vi "Associate Instruments to Paths.vi"(0 "Vector Path Group in":refnum<class "Vector Path Group.lvclass">, 5 "TSM Context":T1, 11 "error in (no error)":errorcluster) -> (4 "Vector Path Group out":refnum<class "Vector Path Group.lvclass">, 15 "error out":errorcluster)   [LabVIEW 2023, in "RFFixtureCharact.Public.lvlib" / "Vector Path Group.lvclass"]
uses:
  Vector Path Group.lvclass
  C:/rfcal/AuxTools/STSRFFixtureCharactUtility/Source/Code Modules/Common/Base Classes/Path Group/Path Group.lvclass
  <vilib>/NI_TestStand_SemiconductorModule/NI_TestStand_Semiconductor_Module.lvlibp/PinMap/General/SemiconductorModuleContext.ctl
  Instruments/Cal Standard/Cal Standard Base/Cal Standard Base.lvclass/Cal Standard Base.ctl
  Charact Result Accessor/Vector/Vector Charact Result Accessor.lvclass
  C:/rfcal/AuxTools/STSRFFixtureCharactUtility/Source/Code Modules/Fixture/Public/Charact Result Accessor/Base/Charact Result Accessor.lvclass
  C:/rfcal/AuxTools/STSRFFixtureCharactUtility/Source/Code Modules/Common/Result Accessor/Result Accessor.lvclass
  Vector Abstract Path/Vector Abstract Path.lvclass/Vector Abstract Path.ctl
  Common/Base Classes/Path/Path.lvclass/Path.ctl
  Vector Abstract Path/Properties/Write Cal Standard Port.vi
  Common/Base Classes/Path/Properties/Read Interval.vi
  Instruments/Cal Standard/Cal Standard Base/Properties/Read Path Connection Map.vi
  Instruments/Cal Standard/Cal Standard Base/Properties/Write Path Connection Map.vi
  Common/Base Classes/Path/Path.lvclass
  Instruments/Cal Standard/Cal Standard Base/Cal Standard Base.lvclass
  Vector Path Group.lvclass/Vector Path Group.ctl
  Common/Base Classes/Path Group/Path Group.lvclass
  <vilib>/NI_TestStand_SemiconductorModule/NI_TestStand_Semiconductor_Module.lvlibp
  Instruments/Cal Standard/Cal Standard Factory/Cal Standard Factory.lvclass
  Vector Abstract Path/Vector Abstract Path.lvclass
  Common/RFCalAndFixtureCharact.Common.lvlib
  <vilib>/addons/_RFCalAndCharactDatabase/NI_RFCalAndCharact_Database_API.lvlibp/Characterization/Characterization.lvlib
  Vector Path/Vector Path.lvclass
  C:/rfcal/AuxTools/STSRFFixtureCharactUtility/Source/Code Modules/Fixture/Public/Charact Result Accessor/Vector/Vector Charact Result Accessor.lvclass
  C:/rfcal/AuxTools/STSRFFixtureCharactUtility/Source/Code Modules/Fixture/Public/Base Classes/Vector/Vector Abstract Path/Vector Abstract Path.lvclass
  C:/rfcal/AuxTools/STSRFFixtureCharactUtility/Source/Code Modules/Common/Base Classes/Path/Path.lvclass
  C:/rfcal/AuxTools/STSRFFixtureCharactUtility/Source/Code Modules/Fixture/Public/Base Classes/Vector/Vector Path/Vector Path.lvclass
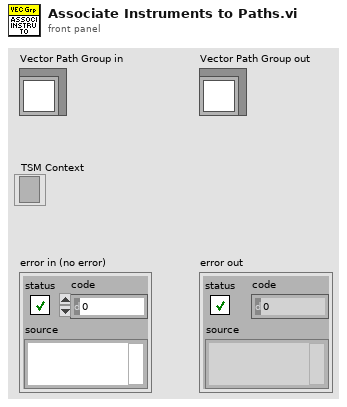
[diagram p1: front panel]
types:
  T1 = typedef "NI_TestStand_Semiconductor_Module.lvlibp/SemiconductorModuleContext.ctl" = refnum<k7>
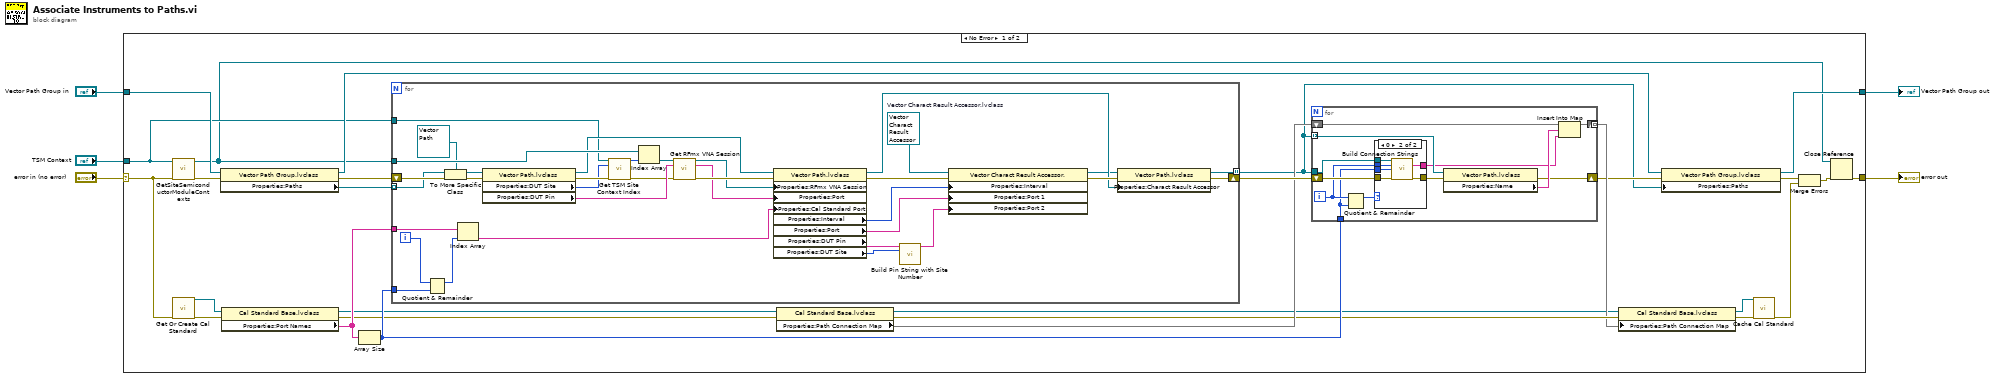
[diagram p0: block diagram]
diagram:
  n1 = case shown="No Error" "error in (no error)" {
    selector: "error in (no error)" -> [w7 w88]
    tunnel: "TSM Context" -> [w28 _]
    tunnel: "Vector Path Group in" -> [w30 w87]
    tunnel: [w29 w88] -> w2
    tunnel: [w31 w87] -> w1
    frame No Error {
      n2 = call <vilib>:"GetSiteSemiconductorModuleContexts.vi"("error in (no error)"=w7, "Semiconductor Module Context"=w28) -> ("error out"=w33:errorcluster, "Site Semiconductor Module Contexts"=w21:T1[])  [unwired: 8 in]
      n3 = call "Get Or Create Cal Standard.vi"("error in (no error)"=w7) -> ("Cal Standard Base out"=w24:refnum<class "Cal Standard Base.lvclass">, "error out"=w25:errorcluster)  [unwired: 13 in]
      n4 = property class="Vector Path Group.lvclass"(reference=w30, error in=w33) -> (reference out=w32:refnum<class "Vector Path Group.lvclass">, error out=w6:errorcluster, "Properties:Paths"=w22:refnum<class "Path.lvclass">[])
      n5 = property class="Cal Standard Base.lvclass"(reference=w24, error in=w25) -> (reference out=w18:refnum<class "Cal Standard Base.lvclass">, error out=w17:errorcluster, "Properties:Port Names"=w23:string[])
      n6 = Array Size(array=w23) -> (size(s)=w19:i32)
      n7 = for {
        tunnel: w21 -> [w86]
        tunnel: w22 -> [w80] mode=indexing
        tunnel: [w64] -> w8 mode=indexing
        tunnel: w28 -> [w74]
        shift-right: [w65] -> w20
        shift-left: w6 -> [w82]
        tunnel: w19 -> [w69]
        tunnel: w23 -> [w72]
        i -> [w68]
        w55 = refnum<class "Vector Charact Result Accessor.lvclass"> refnum  # Vector Charact Result Accessor.lvclass
        n8 = Quotient & Remainder(x=w68, y=w69) -> (x-y*floor(x/y)=w70:i32)  [unwired: 1 out]
        n9 = To More Specific Class(target class=refnum<class "Vector Path.lvclass"> refnum ("STS Vector Fixture Charact.lvlib:Vector Path.lvclass"), reference=w80, error in=w82) -> (specific class reference=w79:refnum<class "Vector Path.lvclass">, error out=w81:errorcluster)
        n10 = Index Array(array=w72, index=w70) -> (element=w62:string)
        n11 = property class="Vector Path.lvclass"(reference=w79, error in=w81) -> (reference out=w83:refnum<class "Vector Path.lvclass">, error out=w84:errorcluster, "Properties:DUT Site"=w76:i32, "Properties:DUT Pin"=w78:string)
        n12 = call "Get TSM Site Context Index.vi"("Semiconductor Module Context"=w74, "Site Number"=w76, "error in (no error)"=w84) -> ("index of Site TSM Context"=w75:i32, "error out"=w77:errorcluster)  [unwired: 11 in]
        n13 = Index Array(array=w86, index=w75) -> (element=w85:T1)
        n14 = call "Get RFmx VNA Session.vi"("TSM Context"=w85, "Pin"=w78, "error in"=w77) -> ("RFmx VNA Session"=w60:refnum<k21>, "Port"=w61:string, "error out"=w73:errorcluster)  [unwired: 10 in]
        n15 = property class="Vector Path.lvclass"(reference=w83, error in=w73, "Properties:RFmx VNA Session"=w60, "Properties:Port"=w61, "Properties:Cal Standard Port"=w62) -> (reference out=w63:refnum<class "Vector Path.lvclass">, error out=w56:errorcluster, "Properties:Interval"=w53:i32, "Properties:Port"=w54:string, "Properties:DUT Pin"=w59:string, "Properties:DUT Site"=w58:i32)
        n16 = call <vilib>:"Build Pin String with Site Number.vi"("Pin Name"=w59, "Site Number"=w58) -> ("Pin String"=w57:string)  [unwired: 13 in]
        n17 = property class="Vector Charact Result Accessor."(reference=w55, error in=w56, "Properties:Interval"=w53, "Properties:Port 1"=w54, "Properties:Port 2"=w57) -> (reference out=w66:refnum<class "Vector Charact Result Accessor.lvclass">, error out=w67:errorcluster)
        n18 = property class="Vector Path.lvclass"(reference=w63, error in=w67, "Properties:Charact Result Accessor"=w66) -> (reference out=w64:refnum<class "Vector Path.lvclass">, error out=w65:errorcluster)
      }
      n19 = property class="Cal Standard Base.lvclass"(reference=w18, error in=w17) -> (reference out=w13:refnum<class "Cal Standard Base.lvclass">, error out=w15:errorcluster, "Properties:Path Connection Map"=w16:map{string, string[]})
      n20 = for {
        shift-right: [w36] -> w9
        shift-left: w20 -> [w45]
        tunnel: w8 -> [w44]
        tunnel: w19 -> [w42]
        tunnel: w8 -> [w40] mode=indexing
        shift-right: [w34] -> w14
        shift-left: w16 -> [w38]
        tunnel: [w34] -> _ mode=indexing
        i -> [w43]
        n21 = Quotient & Remainder(x=w43, y=w42) -> (x-y*floor(x/y)=w41:i32)  [unwired: 1 out]
        n22 = case shown="0" w41 {
          tunnel: [w46 w52] -> w39
          tunnel: w45 -> [w46 w51]
          tunnel: [_ w50] -> w35
          tunnel: w44 -> [_ w49]
          tunnel: w43 -> [_ w48]
          tunnel: w42 -> [_ w47]
          frame Default {
          }
          frame 0 {
            n23 = call "Build Connection Strings.vi"("Vector Paths in"=w49, "Start Index"=w48, "Subgroup Size"=w47, "error in (no error)"=w51) -> ("Connection Strings"=w50:string[], "error out"=w52:errorcluster)  [unwired: 9 in, 1 out]
          }
        }
        n24 = property class="Vector Path.lvclass"(reference=w40, error in=w39) -> (error out=w36:errorcluster, "Properties:Name"=w37:string)  [unwired: 1 out]
        n25 = Insert Into Map(map in=w38, key=w37, value=w35) -> (map out=w34:map{string, string[]})  [unwired: 2 out]
      }
      n26 = property class="Cal Standard Base.lvclass"(reference=w13, error in=w15, "Properties:Path Connection Map"=w14) -> (reference out=w10:refnum<class "Cal Standard Base.lvclass">, error out=w12:errorcluster)
      n27 = property class="Vector Path Group.lvclass"(reference=w32, error in=w9, "Properties:Paths"=w8) -> (reference out=w31:refnum<class "Vector Path Group.lvclass">, error out=w27:errorcluster)
      n28 = call "Cache Cal Standard.vi"("Cal Standard Base in"=w10, "error in (no error)"=w12) -> ("error out"=w11:errorcluster)  [unwired: 12 in, 1 out]
      n29 = Merge Errors(w27, w11) -> (w26:errorcluster)
      n30 = Close Reference(reference=w21, error in (no error)=w26) -> (error out=w29:errorcluster)
    }
    frame Error {
    }
  }
  "error out" <- w2
  "Vector Path Group out" <- w1
